vi "BarPlot-algo.vi"(8 "error in (no error)":errorcluster, 11 "InputData":dbl[](array[numeric])=[20.0, 25.0, 23.0, 26.0]) -> (0 "error out":errorcluster, 3 "Defect Count for Top View":dbl[][](graph))   [LabVIEW 2019, in "Zen Analytics.lvlib" / "Zen Analytics.lvclass"]
uses:
  Zen Analytics.lvclass
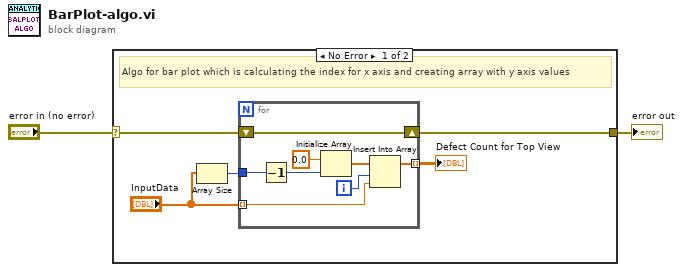
[diagram p0: block diagram]
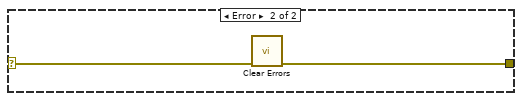
[diagram p2: hidden frame]
diagram:
  n1 = case shown="No Error" "error in (no error)" {
    selector: "error in (no error)" -> [w5 w17]
    tunnel: [w4 w16] -> w1
    frame No Error {
      # "Algo for bar plot which is calculating the index for x axis and creating array with y axis values"
      n2 = Array Size(array="InputData") -> (size(s)=w6:i32)
      n3 = for {
        tunnel: "InputData" -> [w15] mode=indexing
        tunnel: [w13] -> w7 mode=indexing
        tunnel: w6 -> [w10]
        shift-right: [w8] -> w4
        shift-left: w5 -> [w8]
        i -> [w11]
        n4 = Decrement(x=w10) -> (x-1=w9:i32)
        n5 = Initialize Array(0.0 ("element"), w9) -> (w14:dbl[])
        n6 = Insert Into Array(array=w14, index=w11, new element=w15) -> (w13:dbl[])
      }
      "Defect Count for Top View" <- w7
    }
    frame Error {
      n7 = call <vilib>:"Clear Errors.vi"("error in (no error)"=w17) -> ("error out"=w16:errorcluster)  [unwired: 5 in, 1 out]
    }
  }
  "error out" <- w1
